vi "Vbias and Gain Combined Lookup Table dB.vi"() -> (4 "Vbias vs Gain combined dB":dbl[][](array[numeric]), 6 "Gain dB":dbl[](array[numeric]), 8 "Gain Word":u8[](array[numeric]), 10 "Vbias dB":dbl[](array[numeric]), 15 "Vbias Word":u8[](array[numeric]))   [LabVIEW 2020]
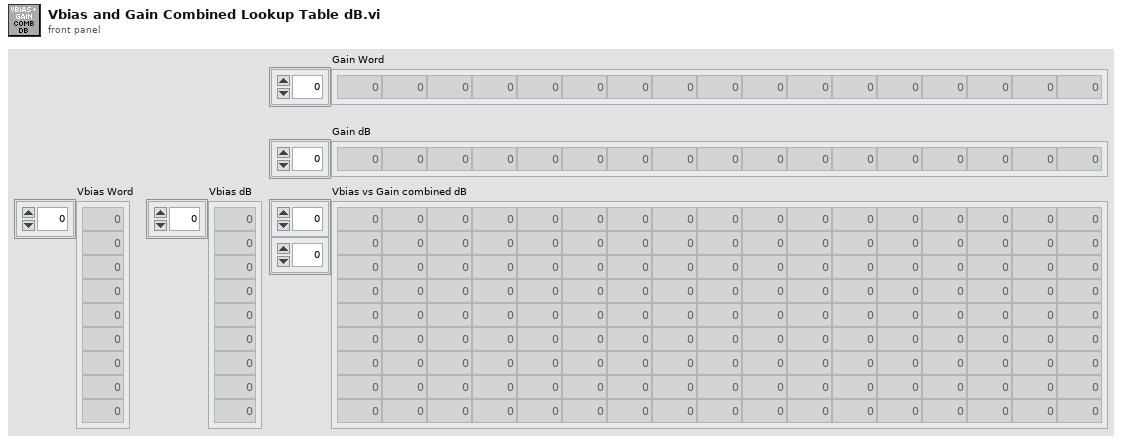
[diagram p1: front panel]
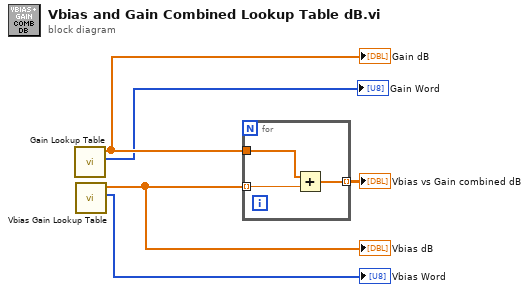
[diagram p0: block diagram]
diagram:
  n1 = call "Gain Lookup Table.vi"() -> ("ROUT<3:0>"=→"Gain Word":u8[], "Gain(dB)"=w3:dbl[])  [unwired: 10 in]
  "Gain dB" <- w3
  n2 = call "Vbias Gain Lookup Table.vi"() -> ("ROUT<7:5>"=→"Vbias Word":u8[], "VB Gain(dB)"=w4:dbl[])  [unwired: 10 in]
  "Vbias dB" <- w4
  n3 = for {
    tunnel: w4 -> [w7] mode=indexing
    tunnel: w3 -> [w8]
    tunnel: [w6] -> w5 mode=indexing
    n4 = Add(x=w8, y=w7) -> (x+y=w6:dbl[])
  }
  "Vbias vs Gain combined dB" <- w5
